vi "stitch interpolated images-ajg.vi"(6 "MAXPICOCOULOMBS":dbl[](array[numeric]), 9 "Calib []":T1, 10 "Array of images to stitch":cluster{u16[][]}[](array[cluster]), 11 "Stitcher in":refnum<class "MagSpecStitcher.lvclass">) -> (2 "stitched array image":dbl[][](graph), 3 "Stitcher out":refnum<class "MagSpecStitcher.lvclass">)   [LabVIEW 2020, in "MagSpecStitcher.lvclass"]
uses:
  MagSpecStitcher/MagSpecStitcher.lvclass
  MagSpecStitcher/subvis/LineoutStatsArray.ctl
  MagSpecStitcher/subvis/LineoutStats.ctl
  MagSpecStitcher/MagSpecStitcher.lvclass/MagSpecStitcher.ctl
  <vilib>/Analysis/1siggen.llb/Ramp Pattern by Samples.vi
  <vilib>/Analysis/8numeric.llb/1D Numeric Integration.vi
  shared/CompressAndUpdate(Poly)/CompressAndUpdate(Numeric).vi
  General GUIs/Device GUIs/GUI_Cameras/color tables/image color table presets.ctl
  <vilib>/Analysis/NI_AALBase.lvlib
  <vilib>/Analysis/NI_AALPro.lvlib
panel:
  in  "Tab Control":enum32{"Maiin", "Page 2", "calib", "Page 3"}(tab)
  in  "subtract BG":bool
  in  "log 2":bool
  out "ChargeAbove5GeV":dbl(graph)
  out "ChargeAbove1GeV":dbl(graph)
  in  "log":bool
  out "ChargeAbove10GeV":dbl(graph)
  in  "get BG":bool
  out "BG":dbl[][](array[numeric])
  out "charge vs angle":sgl[](graph)
  out "charge vs energy":sgl[](graph)
  out "Energy axis":dbl[](array[numeric])
  out "size(s)":i32[](array[numeric])
  out "ysize":dbl
  out "angle axis":dbl[](array[numeric])
  out "x/y":dbl
  out "d theta":dbl
  out "DeltaE":dbl=1.0
  out "index":i32
  out "img pix positions":dbl[](array[numeric])
  out "img sizes reversed":i32[][](array[numeric])
  out "length":i32=11
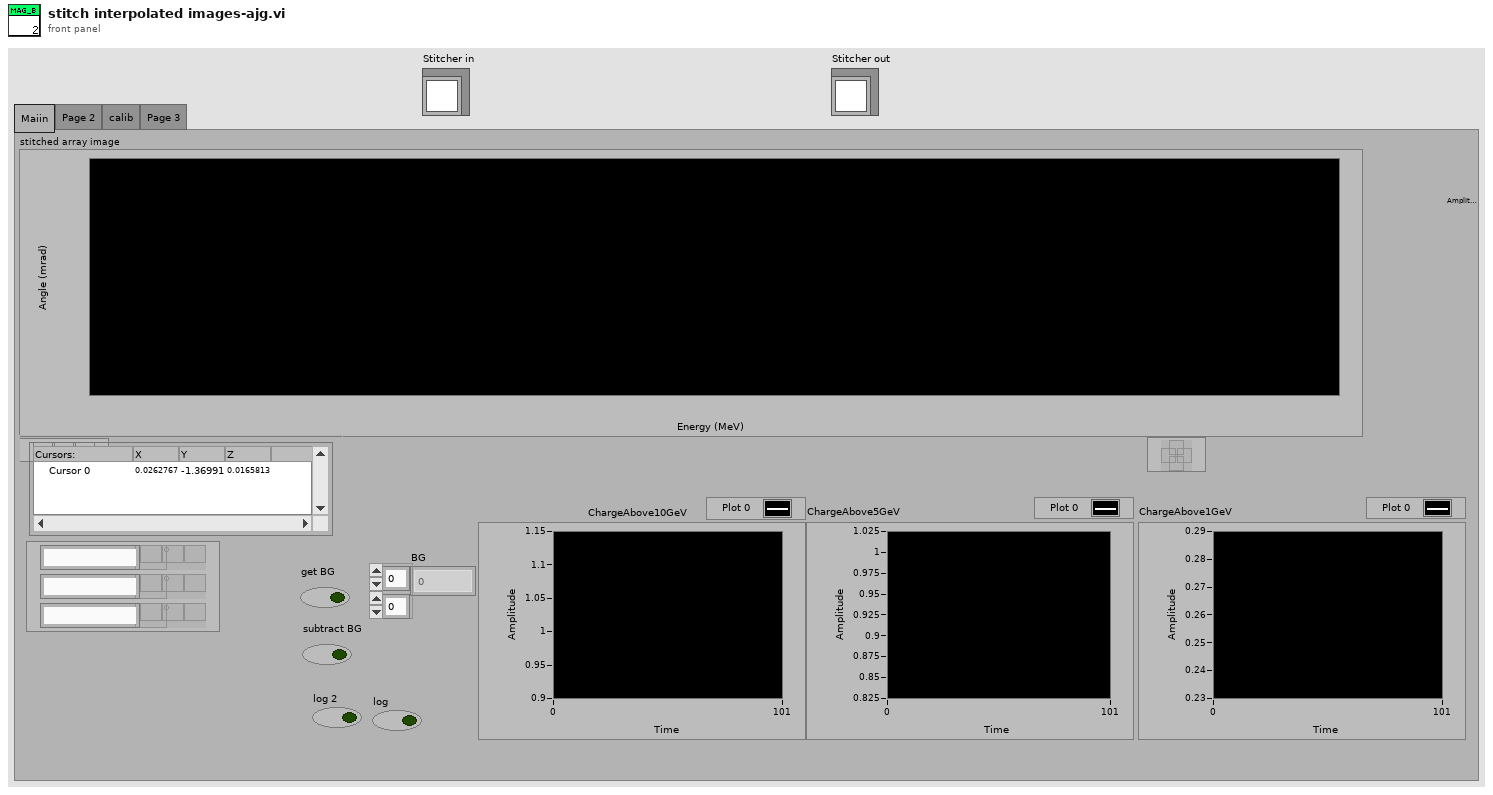
[diagram p1: front panel]
types:
  T1 = typedef "LineoutStatsArray.ctl" = T2[]
  T2 = typedef "LineoutStats.ctl" = cluster{"max X":dbl, "min X":dbl, "Y Size":dbl, "X Size":dbl, "max Y":dbl, "min Y":dbl}
  T3 = enum32{"Invalid", "Standard", "Closed", "Hidden", "Minimized", "Maximized"}
  T4 = typedef "image color table presets.ctl" = enum16{"Greyscale", "Binary", "Gradient", "Rainbow", "Temperature", "enhance low", "blue yellow red", "BYR enhance low", "white blue yellow", "BWR enhance low", "make a new one"}
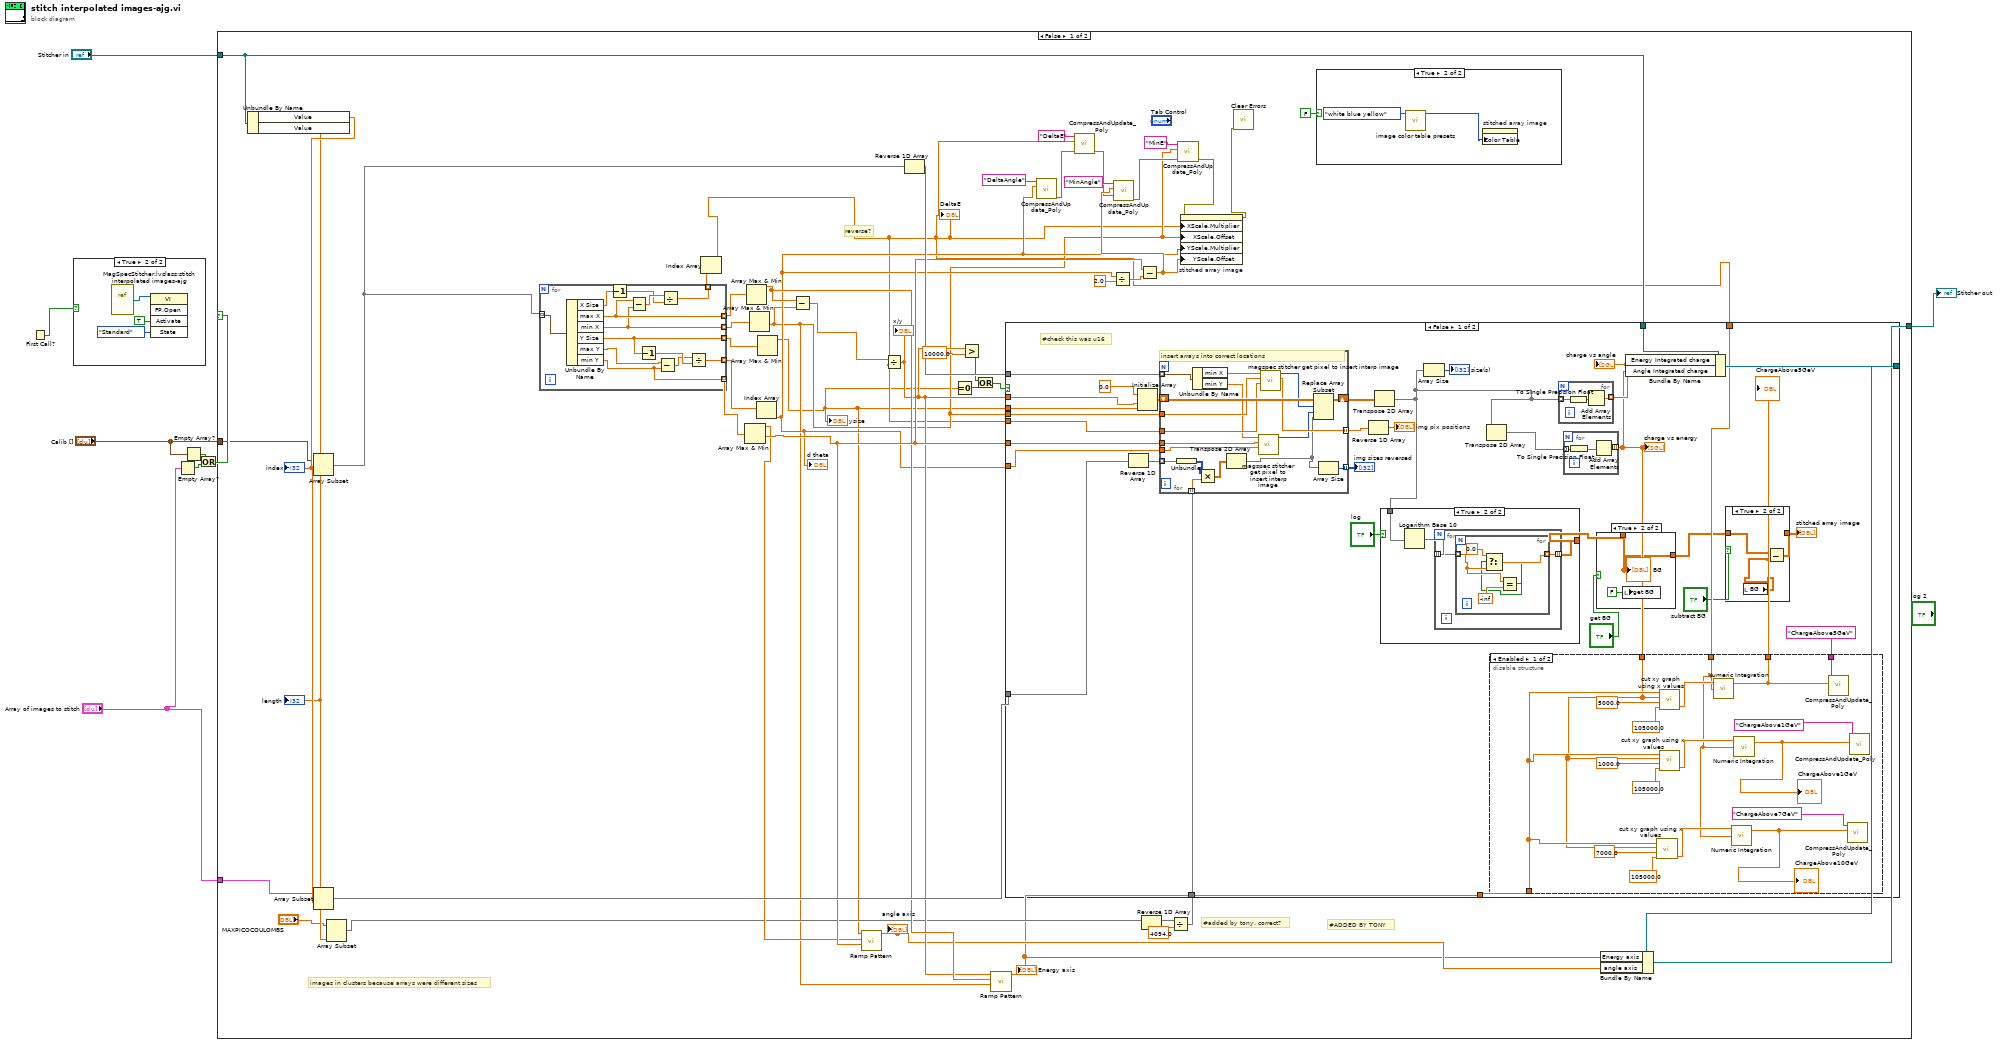
[diagram p0: block diagram]
diagram:
  n1 = First Call?() -> (First Call?: T/F=w1:bool)
  n2 = case shown="True" w1 {
    frame False {
    }
    frame True {
      n3 = vi-ref "MagSpecStitcher.lvclass:stitch interpolated images-ajg.vi"() -> (w11:refnum<vi>)
      n4 = invoke class="VI" method="FP.Open"(reference=w11, "Activate"=TRUE ("Activate?"), "State"=T3."Standard") -> ()  [unwired: 2 in, 5 out]
    }
  }
  n5 = Empty Array?(array="Array of images to stitch") -> (empty?=w4:bool)
  n6 = Empty Array?(array="Calib []") -> (empty?=w5:bool)
  n7 = Or(x=w5, y=w4) -> (x .or. y?=w3:bool)
  n8 = case shown="False" w3 {
    tunnel: "Stitcher in" -> [w31 w170]
    tunnel: "Array of images to stitch" -> [w27 _]
    tunnel: "Calib []" -> [w26 _]
    tunnel: [w25 w170] -> w2
    frame False {
      # "#ADDED BY TONY"
      # "#added by tony. correct?"
      # "reverse?"
      # "images in clusters because arrays were different sizes"
      n9 = Unbundle By Name(w31) -> ("Value"=w30:dbl, "Value"=w21:dbl)
      "index" <- w30
      "length" <- w21
      n10 = Array Subset(array=w26, index=w30, length=w21) -> (w57:T1)
      n11 = Array Subset(array=w27, index=w30, length=w21) -> (w56:cluster{u16[][]}[])
      n12 = Array Subset(array="MAXPICOCOULOMBS", length=w21) -> (w19:dbl[])  [unwired: 1 in]
      n13 = for {
        tunnel: w57 -> [w73] mode=indexing
        tunnel: [w72] -> w48 mode=indexing
        tunnel: [w65] -> w45 mode=indexing
        tunnel: [w71] -> w47 mode=indexing
        tunnel: [w69] -> w46 mode=indexing
        tunnel: [w63] -> w44 mode=indexing
        tunnel: [w62] -> w43 mode=indexing
        n14 = Unbundle By Name(w73) -> ("X Size"=w61:dbl, "max X"=w72:dbl, "min X"=w71:dbl, "Y Size"=w65:dbl, "max Y"=w64:dbl, "min Y"=w62:dbl)
        n15 = Decrement(x=w61) -> (x-1=w68:dbl)
        n16 = Subtract(x=w72, y=w71) -> (x-y=w70:dbl)
        n17 = Decrement(x=w65) -> (x-1=w67:dbl)
        n18 = Subtract(x=w64, y=w62) -> (x-y=w66:dbl)
        n19 = Divide(x=w70, y=w68) -> (x/y=w69:dbl)
        n20 = Divide(x=w66, y=w67) -> (x/y=w63:dbl)
      }
      n21 = Index Array(array=w46) -> (element=w16:dbl)  [unwired: 1 in]
      "DeltaE" <- w16
      n22 = Array Max & Min(array=w43) -> (max value=w51:dbl, min value=w52:dbl)  [unwired: 2 out]
      n23 = Array Max & Min(array=w48) -> (max value=w50:dbl)  [unwired: 3 out]
      n24 = Array Max & Min(array=w47) -> (min value=w18:dbl)  [unwired: 3 out]
      n25 = Index Array(array=w44) -> (element=w37:dbl)  [unwired: 1 in]
      "d theta" <- w37
      n26 = Array Max & Min(array=w45) -> (max value=w12:dbl)  [unwired: 3 out]
      "ysize" <- w12
      n27 = Subtract(x=w50, y=w18) -> (x-y=w60:dbl)
      n28 = call-poly <vilib>:"Ramp Pattern.vi"("start"=w52, "end"=w51, "samples"=w12) -> ("Ramp Pattern"=w29:dbl[])  [unwired: 7 in, 1 out]
      "angle axis" <- w29
      n29 = Divide(x=w60, y=w16) -> (x/y=w49:dbl)
      "x/y" <- w49
      n30 = Reverse 1D Array(array=w57) -> (reversed array=w58:T1)
      n31 = Equal To 0?(x=w12) -> (x = 0?=w13:bool)
      n32 = Greater?(x=w49, y=10000.0) -> (0:w15:bool)
      n33 = Or(x=w15, y=w13) -> (x .or. y?=w14:bool)
      n34 = call-poly <vilib>:"Ramp Pattern.vi"("start"=w18, "end"=w50, "samples"=w49) -> ("Ramp Pattern"=w17:dbl[])  [unwired: 7 in, 1 out]
      "Energy axis" <- w17
      n35 = call-poly "CompressAndUpdate_Poly.vi"("Numeric"=w37, "command or variable name"="DeltaAngle") -> ("error out"=w36:errorcluster)  [unwired: 9 in]
      n36 = call-poly "CompressAndUpdate_Poly.vi"("error in"=w36, "Numeric"=w16, "command or variable name"="DeltaE") -> ("error out"=w35:errorcluster)  [unwired: 8 in]
      n37 = Divide(x=w37, y=2.0) -> (x/y=w53:dbl)
      n38 = Subtract(x=w52, y=w53) -> (x-y=w39:dbl)
      n39 = call-poly "CompressAndUpdate_Poly.vi"("error in"=w35, "Numeric"=w39, "command or variable name"="MinAngle") -> ("error out"=w34:errorcluster)  [unwired: 8 in]
      n40 = Reverse 1D Array(array=w19) -> (reversed array=w23:dbl[])
      n41 = Divide(x=w23, y=4094.0) -> (x/y=w22:dbl[])
      n42 = case shown="False" w14 {
        tunnel: w18 -> [w108 _]
        tunnel: w12 -> [w105 _]
        tunnel: w58 -> [w104 _]
        tunnel: w16 -> [w103 _]
        tunnel: w49 -> [w102 _]
        tunnel: w56 -> [w99 _]
        tunnel: w37 -> [w96 _]
        tunnel: w52 -> [w97 _]
        tunnel: w31 -> [w91 w169]
        tunnel: [w89 w169] -> w28
        tunnel: w22 -> [w88 _]
        tunnel: w17 -> [w85 _]
        tunnel: w16 -> [w83 _]
        frame False {
          # "#check this was u16"
          n43 = Reverse 1D Array(array=w99) -> (reversed array=w107:cluster{u16[][]}[])
          n44 = Initialize Array(sgl 0.0, w102, w105) -> (w106:sgl[][])
          n45 = for {
            tunnel: w103 -> [w166]
            shift-right: [w165] -> w93
            shift-left: w106 -> [w168]
            tunnel: w107 -> [w167] mode=indexing
            tunnel: w108 -> [w159]
            tunnel: w104 -> [w163] mode=indexing
            tunnel: [w161] -> w101 mode=indexing
            tunnel: [w160] -> w100 mode=indexing
            tunnel: w97 -> [w157]
            tunnel: w96 -> [w156]
            tunnel: w88 -> [w154] mode=indexing
            # "insert arrays into correct locations"
            n46 = Unbundle(w167) -> (w151:u16[][])
            n47 = Unbundle By Name(w163) -> ("min X"=w162:dbl, "min Y"=w158:dbl)
            n48 = Multiply(x=w151, y=w154) -> (x*y=w153:dbl[][])
            n49 = Transpose 2D Array(2D array=w153) -> (transposed array=w152:dbl[][])
            n50 = call "magspec stitcher get pixel to insert interp image.vi"("Delta"=w156, "min X of all"=w157, "min X of current"=w158) -> ("X pixel to insert into"=w155:i32)  [unwired: 7 in, 1 out]
            n51 = call "magspec stitcher get pixel to insert interp image.vi"("Delta"=w166, "min X of all"=w159, "min X of current"=w162) -> ("x pixel double prec"=w161:dbl, "X pixel to insert into"=w164:i32)  [unwired: 7 in]
            n52 = Replace Array Subset(array=w168, new element=w152, index (row)=w164, index (col)=w155) -> (w165:sgl[][])
            n53 = Array Size(array=w152) -> (size(s)=w160:i32[])
          }
          "img sizes reversed" <- w100
          n54 = Reverse 1D Array(array=w101) -> (reversed array=→"img pix positions":dbl[])
          n55 = Transpose 2D Array(2D array=w93) -> (transposed array=w82:sgl[][])
          n56 = case shown="True" "log" {
            tunnel: w82 -> [w116 w119]
            tunnel: [w116 w117] -> w77
            frame False {
            }
            frame True {
              n57 = Logarithm Base 10(1:w119) -> (0:w118:sgl[][])
              n58 = for {
                tunnel: w118 -> [w121] mode=indexing
                tunnel: [w120] -> w117 mode=indexing
                n59 = for {
                  tunnel: w121 -> [w123] mode=indexing
                  tunnel: [w125] -> w120 mode=indexing
                  n60 = Equal?(x=w123, y=-inf) -> (x = y?=w122:bool)
                  n61 = Select(t=0.0, s=w122, f=w123) -> (s? t:f=w125:dbl)
                }
              }
            }
          }
          n62 = Array Size(array=w82) -> (size(s)=→"size(s)":i32[])
          n63 = Transpose 2D Array(2D array=w82) -> (transposed array=w92:sgl[][])
          n64 = for {
            tunnel: w82 -> [w149] mode=indexing
            tunnel: [w150] -> w90 mode=indexing
            n65 = To Single Precision Float(number=w149) -> (single precision float=w148:sgl[])
            n66 = Add Array Elements(numeric array=w148) -> (sum=w150:sgl)
          }
          "charge vs angle" <- w90
          n67 = for {
            tunnel: w92 -> [w146] mode=indexing
            tunnel: [w147] -> w84 mode=indexing
            n68 = To Single Precision Float(number=w146) -> (single precision float=w145:sgl[])
            n69 = Add Array Elements(numeric array=w145) -> (sum=w147:sgl)
          }
          "charge vs energy" <- w84
          n70 = disable-structure shown="Enabled" {
            disable-tunnel: "ChargeAbove5GeV" ("command or variable name") -> [w141 _]
            disable-tunnel: [w140 _] -> w86
            disable-tunnel: w85 -> [w128 _]
            disable-tunnel: w84 -> [w127 _]
            disable-tunnel: w83 -> [w129 _]
            frame Enabled {
              n71 = call "cut xy graph using x values.vi"("x_max"=sgl 105000.0, "x_min"=sgl 7000.0, "f(x)"=w127, "x"=w128) -> ("y_cut"=w131:dbl[])  [unwired: 2 out]
              n72 = call "cut xy graph using x values.vi"("x_max"=sgl 105000.0, "x_min"=sgl 5000.0, "f(x)"=w127, "x"=w128) -> ("y_cut"=w142:dbl[])  [unwired: 2 out]
              n73 = call "cut xy graph using x values.vi"("x_max"=sgl 105000.0, "x_min"=sgl 1000.0, "f(x)"=w127, "x"=w128) -> ("y_cut"=w139:dbl[])  [unwired: 2 out]
              n74 = call-poly <vilib>:"Numeric Integration.vi"("dt"=w129, "Input Array"=w142) -> ("result"=w140:dbl)  [unwired: 1 in, 1 out]
              n75 = call-poly <vilib>:"Numeric Integration.vi"("dt"=w129, "Input Array"=w131) -> ("result"=w134:dbl)  [unwired: 1 in, 1 out]
              "ChargeAbove10GeV" <- w134
              n76 = call-poly <vilib>:"Numeric Integration.vi"("dt"=w129, "Input Array"=w139) -> ("result"=w135:dbl)  [unwired: 1 in, 1 out]
              "ChargeAbove1GeV" <- w135
              n77 = call-poly "CompressAndUpdate_Poly.vi"("Numeric"=w140, "command or variable name"=w141) -> ()  [unwired: 9 in, 1 out]
              n78 = call-poly "CompressAndUpdate_Poly.vi"("Numeric"=w134, "command or variable name"="ChargeAbove7GeV") -> ()  [unwired: 9 in, 1 out]
              n79 = call-poly "CompressAndUpdate_Poly.vi"("Numeric"=w135, "command or variable name"="ChargeAbove1GeV") -> ()  [unwired: 9 in, 1 out]
            }
            frame Disabled {
            }
          }
          "ChargeAbove5GeV" <- w86
          n80 = case shown="True" "get BG" {
            tunnel: w77 -> [w109 w110]
            tunnel: [w109 w110] -> w76
            frame False {
            }
            frame True {
              n81 = local write "get BG"(FALSE ("get BG")) -> ()
              "BG" <- w110
            }
          }
          n82 = Bundle By Name(cluster=w91, "Energy Integrated charge"=w90, "Angle Integrated charge"=w84) -> (w89:refnum<class "MagSpecStitcher.lvclass">)
          n83 = case shown="True" "subtract BG" {
            tunnel: w76 -> [w112 w115]
            tunnel: [w112 w114] -> w80
            frame False {
            }
            frame True {
              n84 = local read "BG"() -> (w113:dbl[][])
              n85 = Subtract(x=w115, y=w113) -> (x-y=w114:dbl[][])
            }
          }
          "stitched array image" <- w80
        }
        frame True {
        }
      }
      n86 = call-poly "CompressAndUpdate_Poly.vi"("error in"=w34, "Numeric"=w18, "command or variable name"="MinE") -> ("error out"=w33:errorcluster)  [unwired: 8 in]
      n87 = property on="stitched array image" class="IntGraph (strict)"(error in=w33, "XScale.Multiplier"=w16, "XScale.Offset"=w18, "YScale.Multiplier"=w37, "YScale.Offset"=w39) -> (error out=w32:errorcluster)  [unwired: 1 in, 1 out]
      n88 = call <vilib>:"Clear Errors.vi"("error in (no error)"=w32) -> ()  [unwired: 5 in, 2 out]
      n89 = case shown="True" FALSE {
        frame False {
        }
        frame True {
          n90 = call "image color table presets.vi"("Color table"=image_color_table_presets."white blue yellow") -> ("white to yellow color table"=w74:u32[])  [unwired: 9 in, 1 out]
          n91 = property on="stitched array image" class="IntGraph (strict)"("Color Table"=w74) -> ()  [unwired: 2 in, 2 out]
        }
      }
      n92 = Bundle By Name(cluster=w28, "Energy axis"=w17, "angle axis"=w29) -> (w25:refnum<class "MagSpecStitcher.lvclass">)
    }
    frame True {
    }
  }
  "Stitcher out" <- w2
